vi "IMAQ to Py Object.vi"(8 "error in (no error)":errorcluster, 10 "Image In":T1, 11 "Session Handle in":refnum<data-value>) -> (0 "error out":errorcluster, 2 "Python Object Refnum":T2, 3 "Session Handle out":refnum<data-value>)   [LabVIEW 2020, in "G-Embedded-Python-Interpreter-Toolkit-IMAQ.lvlib"]
uses:
  G-Embedded-Python-Interpreter-Toolkit-IMAQ.lvlib
  G-Embedded-Python-Interpreter-Toolkit/G-Embedded-Python-Interpreter-Toolkit.lvlib
  G-Embedded-Python-Interpreter-Toolkit/IMAQ Image Pointer.ctl
  22f05568-5bba-4402-9e98-aca160827363.vi
  G-Embedded-Python-Interpreter-Toolkit/Python Object Type.ctl
  G-Embedded-Python-Interpreter-Toolkit/Python Object Reference.ctl
  <vilib>/vision/Image Controls.llb/IMAQ Image.ctl
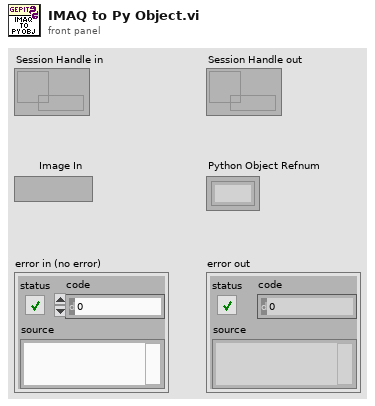
[diagram p1: front panel]
types:
  T1 = typedef "IMAQ Image.ctl" = refnum<image>
  T2 = typedef "G-Embedded-Python-Interpreter-Toolkit.lvlib/Python Object Reference.ctl" = refnum<k1>
  T3 = enum32{"Map Pixel Pointer", "Unmap Pixel Pointer", "Get Pixels Infos"}
  T4 = typedef "G-Embedded-Python-Interpreter-Toolkit.lvlib/IMAQ Image Pointer.ctl" = cluster{"Pixel Pointer":u64, "Line Width":i32, "Width":i32, "Height":i32, "IMAQ Type":u32}
  T5 = typedef "Image Type" = u32
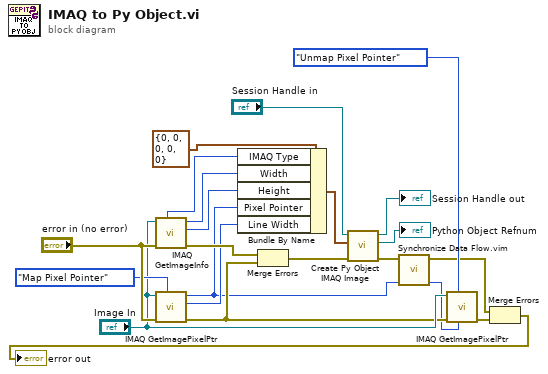
[diagram p0: block diagram]
diagram:
  n1 = call "IMAQ GetImageInfo"("error in (no error)"="error in (no error)", "Image"="Image In") -> ("error out"=w17:errorcluster, "Y Resolution"=w13:i32, "X Resolution"=w14:i32, "Image Type"=w15:T5)  [unwired: 2 in, 4 out]
  n2 = call "IMAQ GetImagePixelPtr"("Function"=T3."Map Pixel Pointer", "error in (no error)"="error in (no error)", "Image"="Image In") -> ("error out"=w7:errorcluster, "LineWidth(Pixels)"=w12:i32, "Pixel Pointer out"=w3:u64)  [unwired: 3 in, 3 out]
  n3 = Bundle By Name(cluster=T4 {"Pixel Pointer"=0, "Line Width"=0, "Width"=0, "Height"=0, "IMAQ Type"=0} ("IMAQ Pointer"), "IMAQ Type"=w15, "Width"=w14, "Height"=w13, "Pixel Pointer"=w3, "Line Width"=w12) -> (w16:T4)
  n4 = Merge Errors(w17, w7) -> (w11:errorcluster)
  n5 = call "Create Py Object IMAQ Image.vi"("error in (no error)"=w11, "IMAQ Pointer"=w16, "Session Handle in"="Session Handle in") -> ("error out"=w9:errorcluster, "Python Object Refnum"=→"Python Object Refnum":T2, "Session Handle out"=→"Session Handle out":refnum<data-value>)  [unwired: 6 in]
  n6 = call "Synchronize Data Flow.vim"("input 4"=w3, "input 1"=w9) -> ("output 4"=w2:u64, "output 1"=w5:errorcluster)  [unwired: 2 in, 2 out]
  n7 = call "IMAQ GetImagePixelPtr"("Pixel Pointer in"=w2, "Function"=T3."Unmap Pixel Pointer", "error in (no error)"=w7, "Image"="Image In") -> ("error out"=w4:errorcluster)  [unwired: 2 in, 5 out]
  n8 = Merge Errors(w5, w4) -> (→"error out":errorcluster)
